vi "R1C_TX_Att0.vi"() -> ()   [LabVIEW 2018]
uses:
  Types/Att(0-0.5-31.5).ctl
  Types/RFU.ctl
  Types/RF.ctl
panel:
  out "Error_Out":errorcluster
  out "VISA_Rsrc_Out":refnum<visa-resource-name>
  in  "RF":T1 items=["RF_0", "RF_1", "RF_2", "RF_3"]
  in  "RFU":T2
  in  "Error_In":errorcluster
  in  "Auto_Sel_Rsrc?":bool=TRUE
  in  "Att":T3 items=["0.0", "0.5", "1.0", "1.5", "2.0", "2.5", "3.0", "3.5", "4.0", "4.5", "5.0", "5.5", "6.0", "6.5", "7.0", "7.5", "8.0", "8.5", "9.0", "9.5", "10.0", "10.5", "11.0", "11.5", "12.0", "12.5", "13.0", "13.5", "14.0", "14.5", "15.0", "15.5", "16.0", "16.5", "17.0", "17.5", "18.0", "18.5", "19.0", "19.5", "20.0", "20.5", "21.0", "21.5", "22.0", "22.5", "23.0", "23.5", "24.0", "24.5", "25.0", "25.5", "26.0", "26.5", "27.0", "27.5", "28.0", "28.5", "29.0", "29.5", "30.0", "30.5", "31.0", "31.5"]
  in  "VISA_Rsrc_In":refnum<visa-resource-name>
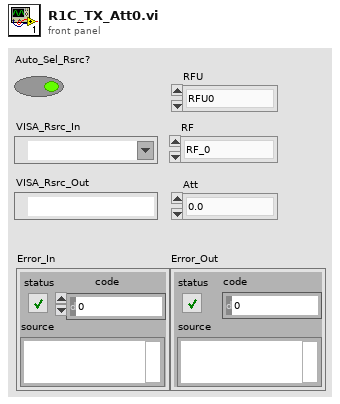
[diagram p1: front panel]
types:
  T1 = typedef "RF.ctl" = u16
  T2 = typedef "RFU.ctl" = enum8{"RFU0", "RFU1", "RFU2", "RFU3", "RFU4"}
  T3 = typedef "Att(0-0.5-31.5).ctl" = dbl
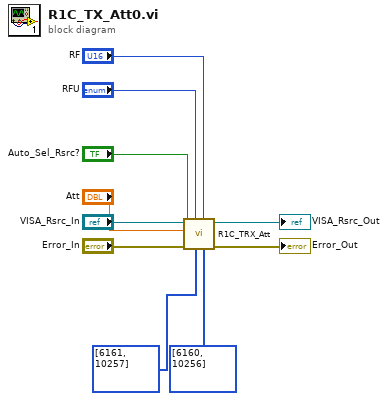
[diagram p0: block diagram]
diagram:
  n1 = call "R1C_TRX_Att.vi"("Offset_Idle_OP"=u32[] [6160, 10256] ("Offset"), "RF"="RF", "Offset_Reg_Data"=u32[] [6161, 10257] ("Offset"), "RFU"="RFU", "Error_In"="Error_In", "Auto_Sel_Rsrc?"="Auto_Sel_Rsrc?", "Att"="Att", "VISA_Rsrc_In"="VISA_Rsrc_In") -> ("Error_Out"=→"Error_Out":errorcluster, "VISA_Rsrc_Out"=→"VISA_Rsrc_Out":refnum<visa-resource-name>)  [unwired: 2 in]
